vi "Select Custom Device.vi"(9 "Main GUID":string="8dfd0406-1a5d-45dd-a1d7-1d4d9090bfa4", 10 "CD Path":string, 11 "NIVS.System Definition Root":refnum<k24>) -> (1 "Cancelled?":bool, 2 "IP Address":string="Targets/Controller/Custom Devices/Communication Example", 3 "Custom Device Path Out":string="Targets/Controller/Custom Devices/Communication Example")   [LabVIEW 2013, in "PID Control Workspace Tool.lvlib"]
uses:
  PID Control Workspace Tool.lvlib
  NationalInstruments.VeriStand.SystemStorage
panel:
  in  "Cancel":bool
  in  "Select":bool
  in  "Custom Device Path":string(tree)
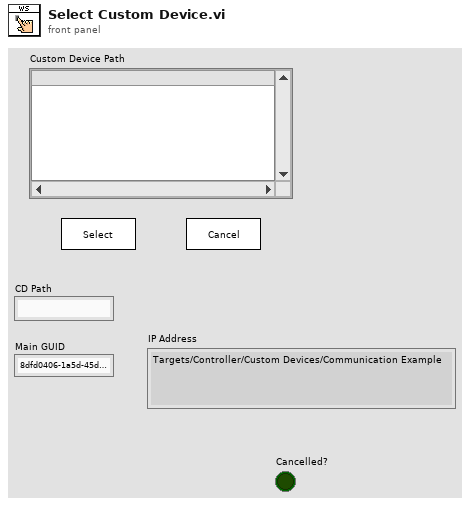
[diagram p1: front panel]
types:
  T1 = enum8{"Enabled", "Disabled", "Disabled and Grayed Out"}
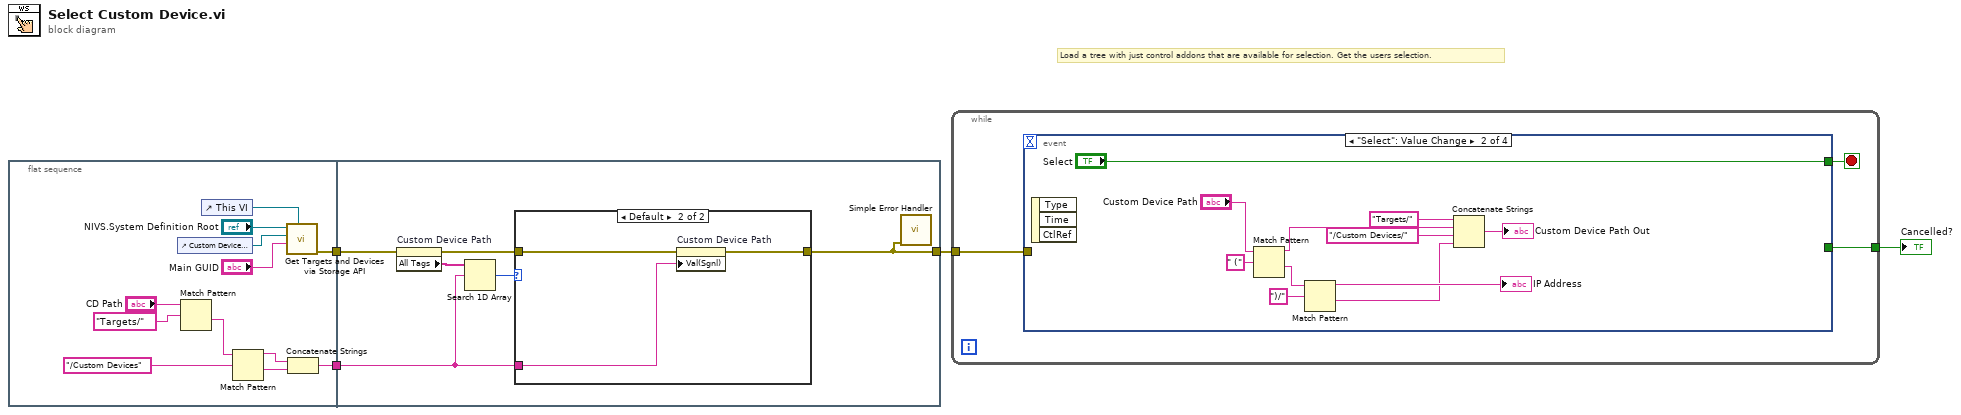
[diagram p0: block diagram]
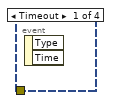
[diagram p2: hidden frame]
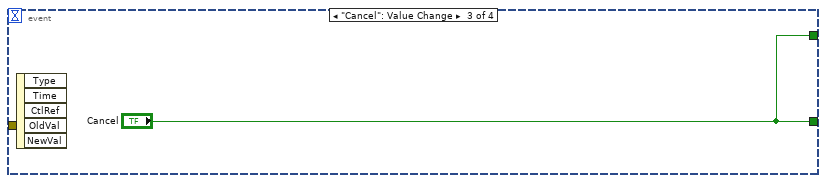
[diagram p3: hidden frame]
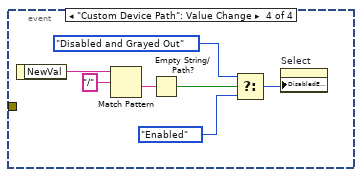
[diagram p4: hidden frame]
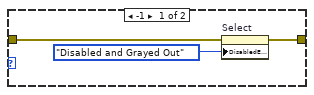
[diagram p5: hidden frame]
diagram:
  # "Load a tree with just control addons that are available for selection. Get the users selection."
  n1 = flat-sequence {
    tunnel: [w13] -> w3
    tunnel: [w5] -> w1
    tunnel: [w22] -> w4
    tunnel: w3 -> [w21]
    tunnel: w1 -> [w18]
    frame #0 {
      n2 = control-ref of="Custom Device Path"() -> (w15:refnum<vi>)
      n3 = Match Pattern(string="CD Path", regular expression="Targets/") -> (after substring=w8:string)  [unwired: 1 in, 3 out]
      n4 = control-ref of="This VI"() -> (w12:refnum<vi>)
      n5 = Match Pattern(string=w8, regular expression="/Custom Devices") -> (before substring=w10:string, after substring=w11:string)  [unwired: 1 in, 2 out]
      n6 = call "Get Targets and Devices via Storage API.vi"("VI reference (current VI)"=w12, "Main GUID"="Main GUID", "Tree"=w15, "NIVS.System Definition Root"="NIVS.System Definition Root") -> ("error out"=w13:errorcluster)  [unwired: 6 in, 1 out]
      n7 = Concatenate Strings(w10, w11) -> (w5:string)
    }
    frame #1 {
      n8 = property on="Custom Device Path" class="Tree (strict)"(error in=w21) -> (error out=w20:errorcluster, "All Tags"=w19:string[])  [unwired: 1 in, 1 out]
      n9 = Search 1D Array(1D array=w19, element=w18) -> (index of element=w17:i32)  [unwired: 1 in]
      n10 = case shown="Default" w17 {
        tunnel: [w25 w28] -> w22
        tunnel: w20 -> [w24 w27]
        tunnel: w18 -> [_ w26]
        frame -1 {
          n11 = property on="Select" class="Bool"(error in=w24, "DisabledEnum"=T1."Disabled and Grayed Out" ("Disabled")) -> (error out=w25:errorcluster)  [unwired: 1 in, 1 out]
        }
        frame Default {
          n12 = property on="Custom Device Path" class="Tree (strict)"(error in=w27, "Val(Sgnl)"=w26) -> (error out=w28:errorcluster)  [unwired: 1 in, 1 out]
        }
      }
      n13 = call <vilib>:"Simple Error Handler.vi"("error in (no error)"=w22) -> ()  [unwired: 4 in, 5 out]
    }
  }
  n14 = while {
    tunnel: w4 -> [w31]
    tunnel: [w29] -> w2
    stop <- w30 stop-if-true
    n15 = event shown="[1] \"Select\": Value Change" {
      selector: _ -> [_ _ _ _]
      dyn-events: _ -> [_ _ _ _]
      timeout: _ -> [_ _ _ _]
      tunnel: w31 -> [_ _ _ _]
      tunnel: [_ "Select" "Cancel" _] -> w30
      tunnel: [_ _ "Cancel" _] -> w29
      event Timeout {
        n16 = event-data() -> ()  [unwired: 1 in, 2 out]
      }
      event "Select": Value Change {
        n17 = event-data() -> ()  [unwired: 1 in, 3 out]
        n18 = Match Pattern(string="Custom Device Path", regular expression=" (") -> (before substring=w33:string, after substring=w36:string)  [unwired: 1 in, 2 out]
        n19 = Match Pattern(string=w36, regular expression=")/") -> (before substring=→"IP Address":string, after substring=w32:string)  [unwired: 1 in, 2 out]
        n20 = Concatenate Strings("Targets/" ("string"), w33, "/Custom Devices/" ("string"), w32) -> (→"Custom Device Path Out":string)
      }
      event "Cancel": Value Change {
        n21 = event-data() -> ()  [unwired: 1 in, 5 out]
      }
      event "Custom Device Path": Value Change {
        n22 = event-data() -> ("NewVal"=w49:string)  [unwired: 1 in]
        n23 = Match Pattern(string=w49, regular expression="/") -> (after substring=w48:string)  [unwired: 1 in, 3 out]
        n24 = Empty String/Path?(string/path=w48) -> (empty?=w47:bool)
        n25 = Select(t=T1."Disabled and Grayed Out" ("Disabled"), s=w47, f=T1."Enabled" ("Disabled")) -> (s? t:f=w44:T1)
        n26 = property on="Select" class="Bool"("DisabledEnum"=w44) -> ()  [unwired: 2 in, 2 out]
      }
    }
  }
  "Cancelled?" <- w2
